vi "Organize Data With Analog Trigger.vi"(0 "Coefficients":T2, 1 "Trigger Data Index":u32, 5 "System Type":T1, 7 "DAQ":sgl[][](array[numeric]), 9 "Channel Filter":bool[](array[boolean]), 11 "Sensor (scaling)":T3(array[cluster])) -> (4 "Scaled Data":sgl[][](array[numeric]), 6 "trigger data":sgl[](array[numeric]))   [LabVIEW 2023]
uses:
  Type Defs and Controls/Coeffs Cluster Type Def.ctl
  Type Defs and Controls/System Type.ctl
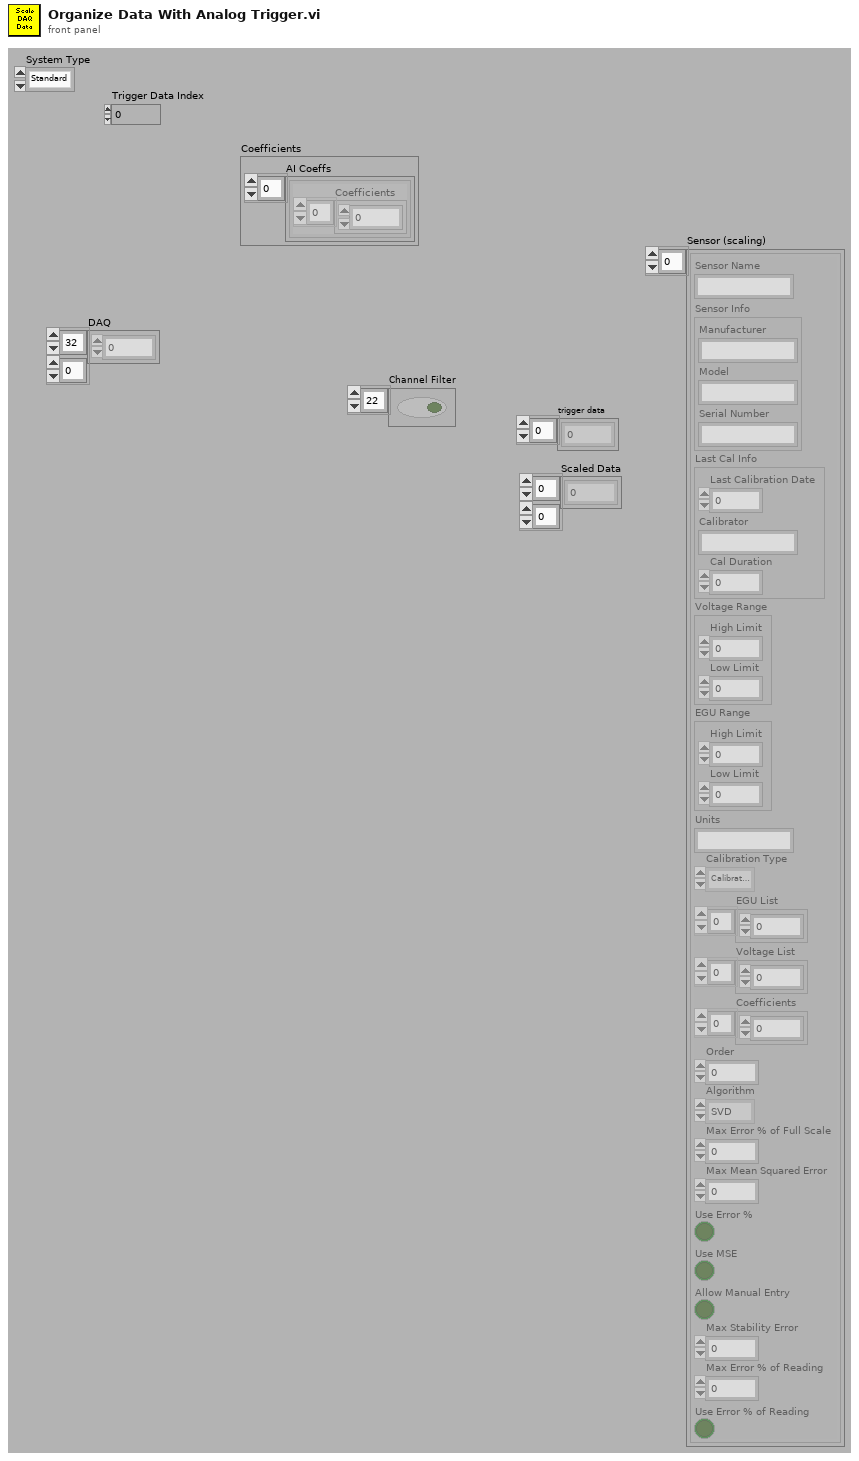
[diagram p1: front panel]
types:
  T1 = typedef "System Type.ctl" = enum16{"Standard", "Deformation", "Standard 8TC"}
  T2 = typedef "Coeffs Cluster Type Def.ctl" = cluster{"AI Coeffs":cluster{"Coefficients":dbl[]}[]}
  T3 = cluster{"Sensor Name":string, "Sensor Info":cluster{"Manufacturer":string, "Model":string, "Serial Number":string}, "Last Cal Info":cluster{"Last Calibration Date":dbl, "Calibrator":string, "Cal Duration":i32}, "Voltage Range":cluster{"High Limit":dbl, "Low Limit":dbl}, "EGU Range":cluster{"High Limit":dbl, "Low Limit":dbl}, "Units":string, "Calibration Type":enum16{"Calibrate Analog", "Compare Analog Calibration"}, "EGU List":dbl[], "Voltage List":dbl[], "Coefficients":dbl[], "Order":i32, "Algorithm":enum32{"SVD", "Givens", "Givens2", "Householder", "LU Decomposition", "Cholesky"}, "Max Error % of Full Scale":dbl, "Max Mean Squared Error":dbl, "Use Error %":bool, "Use MSE":bool, "Allow Manual Entry":bool, "Max Stability Error":dbl, "Max Error % of Reading":dbl, "Use Error % of Reading":bool}[]
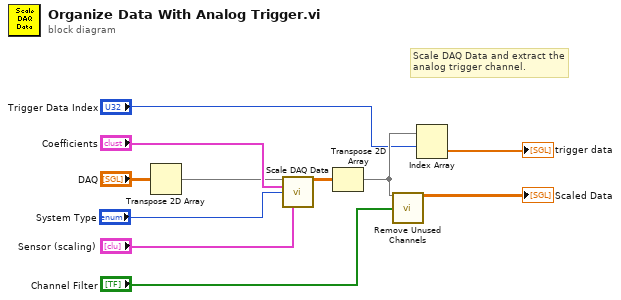
[diagram p0: block diagram]
diagram:
  # "Scale DAQ Data and extract the\nanalog trigger channel."
  n1 = Transpose 2D Array(2D array="DAQ") -> (transposed array=w4:sgl[][])
  n2 = call "Scale DAQ Data.vi"("Data Read"=w4, "Coefficients"="Coefficients", "System Type"="System Type", "Sensor (scaling)"="Sensor (scaling)") -> ("Scaled Data"=w10:sgl[][])  [unwired: 11 in]
  n3 = Transpose 2D Array(2D array=w10) -> (transposed array=w8:sgl[][])
  n4 = call "Remove Unused Channels.vi"("Data in"=w8, "Channel Filter"="Channel Filter") -> ("Data out"=→"Scaled Data":sgl[][])  [unwired: 13 in]
  n5 = Index Array(array=w8, index (row)="Trigger Data Index") -> (element=→"trigger data":sgl[])  [unwired: 1 in]
